vi "_MOV.vi"(0 "System no.":i32=1 min=1 max=4 step=1, 2 "Axes to move":string[](array[string]), 3 "Position values":dbl[](array[numeric]) format="%.6f", 4 "No.of digits":i16=4, 5 "error in":errorcluster) -> (19 "error out":errorcluster)   [LabVIEW 2014]
doc: "Moves specified axes to specified absolute positions. No. of digits is the number of digits after the decimal point in the position value(s) that will be sent.\n\nValid for Analog systems, C-702, C-843, C-843.PM, C-844, C-848, C-865, C-866, C-867, C-880, C-880K005, E-516, E-517, E-710, E-712, E-725, E-753, E-755, E-761, E-816, E-761, F-206, M-8X0, Mercury\n\nC-867: This command works only in closed-loop operation. \nMotion commands like MOV are not allowed when a joystick is active on the axis.\n\nC-880K005: VI only supported when called through PI_Multix.vi\n\nE-517: Motion commands like MOV are not allowed when the E-517 is in OFFLINE mode or when the wave generator output is active. When a macro is running on the E-517, MOV will be executed not until the macro is finished or stopped. See \"Control Value Generation\" and \"Control Modes\" in the E- 517 User manual for details.\n\nE-710: See also \"NMOV.vi\" in \"Old commands.llb\".\n\nE-712: Motion commands are not allowed when a wave generator is active or the analog input is used for target generation.\n\nE-725: Motion commands are not allowed when a wave generator is active or the analog input is used for target generation.\n\nE-753: Motion commands are not allowed when the wave generator is active or the analog input is used for target generation.\n\nE-755: Command not available for E-755.101.\n\nE-816: Only one axis per command allowed. It is necessary to wait a certain time before sending the next command to prevent it from being lost. \n\nE-861: This command works only in closed-loop operation. With open-loop systems, use OAD or OSM instead to command motion. Motion commands like MOV are not allowed when a joystick is active on the axis.\n\nF-206: No mix between F-206 axes X,Y,Z,U,V,W and separate axes A,B allowed"
panel:
  # "Moves stage to absolute position."
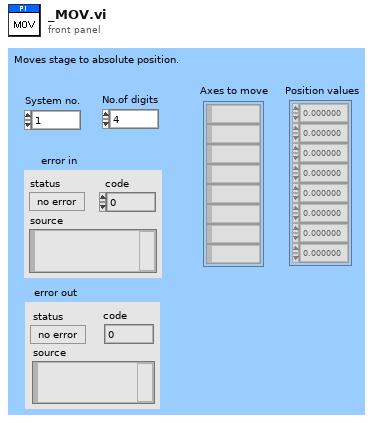
[diagram p1: front panel]
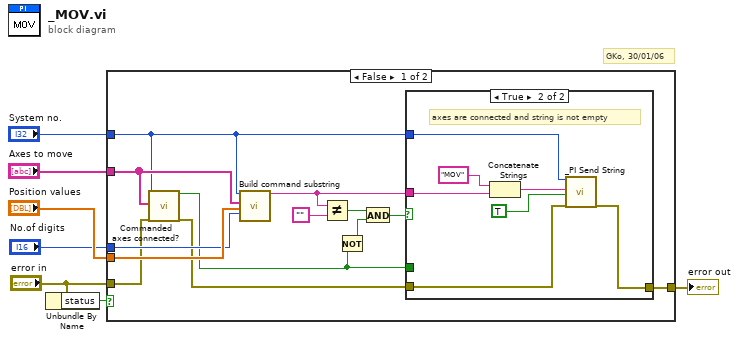
[diagram p0: block diagram]
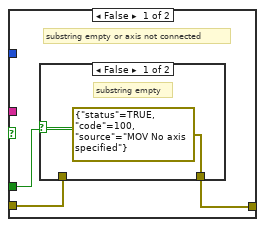
[diagram p2: hidden frame]
diagram:
  # "GKo, 30/01/06"
  n1 = Unbundle By Name("error in") -> ("status"=w1:bool)
  n2 = case shown="False" w1 {
    tunnel: [w20 w33] -> w7
    tunnel: "Position values" -> [w17 _]
    tunnel: "No.of digits" -> [w16 _]
    tunnel: "System no." -> [w8 _]
    tunnel: "Axes to move" -> [w14 _]
    tunnel: "error in" -> [w9 w33]
    frame False {
      n3 = call "Commanded axes connected?.vi"("System no."=w8, "Commanded axes"=w14, "error in"=w9) -> ("Controller error"=w12:bool, "error out"=w15:errorcluster)  [unwired: 15 in]
      n4 = call "Build command substring.vi"("System no."=w8, "Affected axes"=w14, "Parameters"=w17, "No. of digits"=w16) -> ("Command substring"=w18:string)  [unwired: 15 in]
      n5 = Not Equal?(x=w18, y="") -> (x != y?=w13:bool)
      n6 = Not(x=w12) -> (.not. x?=w11:bool)
      n7 = And(x=w13, y=w11) -> (x .and. y?=w10:bool)
      n8 = case shown="True" w10 {
        tunnel: w18 -> [_ w31]
        tunnel: [w23 w27] -> w20
        tunnel: w15 -> [w21 w28]
        tunnel: w12 -> [w22 _]
        tunnel: w8 -> [_ w26]
        frame False {
          # "substring empty or axis not connected"
          n9 = case shown="False" w22 {
            tunnel: [errorcluster {"status"=TRUE, "code"=100, "source"="MOV No axis specified"} ("error out") w25] -> w23
            tunnel: w21 -> [_ w25]
            frame False {
              # "substring empty"
            }
            frame True {
              # "commanded axis not connected"
            }
          }
        }
        frame True {
          # "axes are connected and string is not empty"
          n10 = Concatenate Strings("MOV", w31) -> (w29:string)
          n11 = call "_PI Send String.vi"("System no."=w26, "String to send"=w29, "Attach termination char.?"=TRUE ("Attach Linefeed?"), "error in"=w28) -> ("error out"=w27:errorcluster)  [unwired: 15 in]
        }
      }
    }
    frame True {
    }
  }
  "error out" <- w7
